vi "AlliGator Read IRFs & Fit Data HDF5 File Metadata.vi"(8 "error in (no error)":errorcluster, 11 "ref in":T1 format="%.0x") -> (0 "error out":errorcluster, 1 "File Metadata":string, 3 "ref out":T1 format="%.0x")   [LabVIEW 2021, in "AlliGator Decay Fit Parameter Map.lvlib"]
doc: "Reads Decay Fit Parameter Map metadata from HDF5 file."
uses:
  AlliGator Decay Fit Parameter Map.lvlib
  <vilib>/addons/h5labview2/base/hid_t.ctl
  <vilib>/addons/h5labview2/base/lib_path.vi
  <vilib>/addons/h5labview2/base/H5Equery.vi
  <vilib>/addons/h5labview2/dataset/H5Dread.llb/H5Dread.xnode
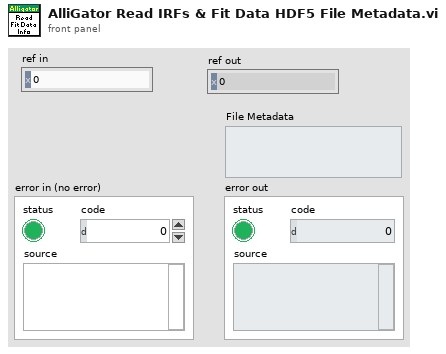
[diagram p1: front panel]
types:
  T1 = typedef "hid_t.ctl" = i64
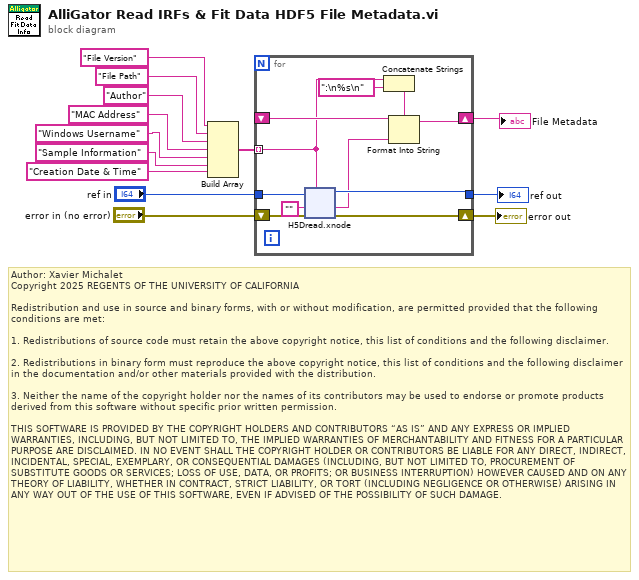
[diagram p0: block diagram]
diagram:
  # "Author: Xavier Michalet\nCopyright 2025 REGENTS OF THE UNIVERSITY OF CALIFORNIA\n\nRedistribution and use in source and binary forms, with or without modification, are permitted provided that the following conditions are met:\n\n1. Redistributions of source code must retain the above copyright notice, this list of conditions and the following disclaimer.\n\n2. Redistributions in binary form must reproduce the above copyright notice, this list of conditions and the following disclaimer in the documentation and/or other materials provided with the distribution.\n\n3. Neither the name of the copyright holder nor the names of its contributors may be used to endorse or promote products derived from this software without specific prior written permission.\n\nTHIS SOFTWARE IS PROVIDED BY THE COPYRIGHT HOLDERS AND CONTRIBUTORS “AS IS” AND ANY EXPRESS OR IMPLIED WARRANTIES, INCLUDING, BUT NOT LIMITED TO, THE IMPLIED WARRANTIES OF MERCHANTABILITY AND FITNESS FOR A PARTICULAR PURPOSE ARE DISCLAIMED. IN NO EVENT SHALL THE COPYRIGHT HOLDER OR CONTRIBUTORS BE LIABLE FOR ANY DIRECT, INDIRECT, INCIDENTAL, SPECIAL, EXEMPLARY, OR CONSEQUENTIAL DAMAGES (INCLUDING, BUT NOT LIMITED TO, PROCUREMENT OF SUBSTITUTE GOODS OR SERVICES; LOSS OF USE, DATA, OR PROFITS; OR BUSINESS INTERRUPTION) HOWEVER CAUSED AND ON ANY THEORY OF LIABILITY, WHETHER IN CONTRACT, STRICT LIABILITY, OR TORT (INCLUDING NEGLIGENCE OR OTHERWISE) ARISING IN ANY WAY OUT OF THE USE OF THIS SOFTWARE, EVEN IF ADVISED OF THE POSSIBILITY OF SUCH DAMAGE."
  n1 = Build Array("File Version" ("dataset name"), "File Path" ("dataset name"), "Author" ("dataset name"), "MAC Address" ("dataset name"), "Windows Username" ("dataset name"), "Sample Information" ("name"), "Creation Date & Time" ("dataset name")) -> (w6:string[])
  n2 = for {
    tunnel: w6 -> [w15] mode=indexing
    shift-right: [w22] -> w3
    shift-left: "error in (no error)" -> [w23]
    shift-right: [w17] -> w2
    shift-left: _ -> [w20]
    tunnel: "ref in" -> [w24]
    tunnel: [w21] -> w4
    n3 = xnode "H5Dread.xnode"("dataset name (this)"=w15, "error in (no error)"=w23, "default"="", "ref in"=w24) -> ("error out"=w22:errorcluster, "data"=w16:string, "ref out"=w21:T1)  [unwired: 2 in, 1 out]
    n4 = Concatenate Strings(w15, ":\n%s\n" ("string")) -> (w18:string)
    n5 = Format Into String(format string=w18, initial string=w20, w16) -> (resulting string=w17:string)  [unwired: 1 in, 1 out]
  }
  "error out" <- w3
  "ref out" <- w4
  "File Metadata" <- w2
